vi "GetTeleopQueue.vi"(8 "error in (no error)":errorcluster) -> (0 "error out":errorcluster, 3 "queue out":refnum<queue>)   [LabVIEW 2013]
doc: "Outputs the teleop queue (of type TeleopInstruction), and opens it if necessary (i.e. in Begin)."
uses:
  TeleopInstruction.ctl
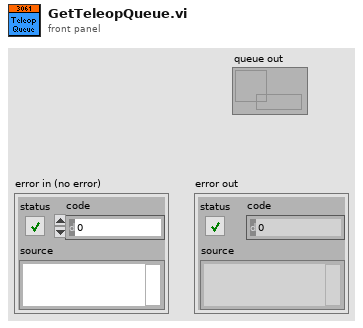
[diagram p1: front panel]
types:
  T1 = typedef "TeleopInstruction.ctl" = cluster{"cDriveLeft":dbl, "cDriveRight":dbl, "cAutoDistance":bool, "cHalfDrive":bool, "cStraightDrive":bool, "cReverseDrive":bool, "cSonicShifter":bool, "cRoller":dbl, "cCollector":dbl, "cCatch":bool, "cCollectorWrap":bool, "cShooter":bool, "cClapper":bool, "cFiringPneumatic":bool, "cKickerPneumatic":bool, "cRollerPneumatic":bool, "TeleopID":i32}
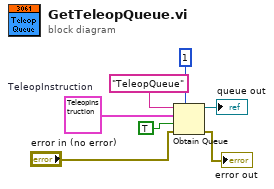
[diagram p0: block diagram]
diagram:
  w3 = T1 {"cDriveLeft"=0.0, "cDriveRight"=0.0, "cAutoDistance"=FALSE, "cHalfDrive"=FALSE, "cStraightDrive"=FALSE, "cReverseDrive"=FALSE, "cSonicShifter"=FALSE, "cRoller"=0.0, "cCollector"=0.0, "cCatch"=FALSE, "cCollectorWrap"=FALSE, "cShooter"=FALSE, "cClapper"=FALSE, "cFiringPneumatic"=FALSE, "cKickerPneumatic"=FALSE, "cRollerPneumatic"=FALSE, "TeleopID"=0}  # TeleopInstruction
  n1 = Obtain Queue(max queue size (-1, unlimited)=1, name (unnamed)="TeleopQueue", element data type=w3, create if not found? (T)=TRUE, error in (no error)="error in (no error)") -> (queue out=→"queue out":refnum<queue>, error out=→"error out":errorcluster)  [unwired: 1 out]
